vi "Prepare Two Step Build.vi"(8 "error in (no error)":errorcluster, 11 "SDIST in":refnum<class "NI_AB_API_SDIST.lvclass">) -> (0 "error out":errorcluster, 2 "Build Context":refnum<vi>, 3 "SDIST out":refnum<class "NI_AB_API_SDIST.lvclass">)   [LabVIEW 2020, in "NI_AB_API_SDIST.lvclass"]
uses:
  <vilib>/AppBuilder/AB_API/SDIST/NI_AB_API_SDIST.lvclass
  <vilib>/AppBuilder/AB_API/Build/NI_AB_API_Build.lvclass
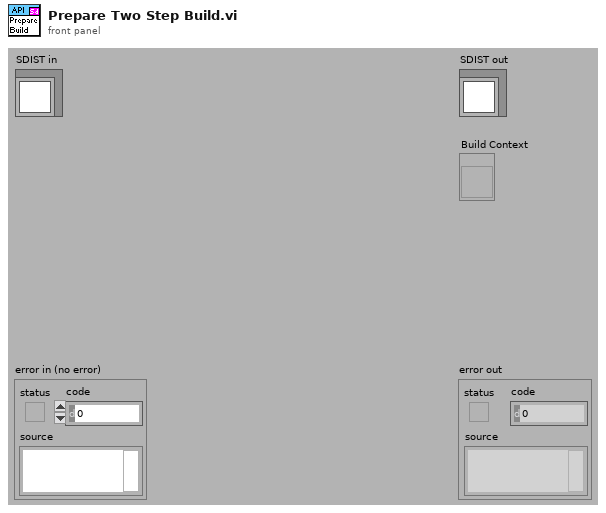
[diagram p1: front panel]
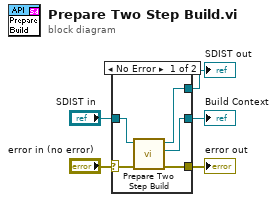
[diagram p0: block diagram]
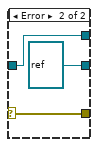
[diagram p2: hidden frame]
diagram:
  n1 = case shown="No Error" "error in (no error)" {
    selector: "error in (no error)" -> [w9 w13]
    tunnel: [w6 w13] -> w4
    tunnel: [w8 w12] -> w2
    tunnel: "SDIST in" -> [w10 w12]
    tunnel: [w7 refnum<vi> refnum ("Build Context")] -> w1
    frame No Error {
      n2 = call-parent "Prepare Two Step Build.vi"("error in (no error)"=w9, "NI_AB_API_Build in"=w10) -> ("error out"=w6:errorcluster, "Build Context"=w7:refnum<vi>, "NI_AB_API_Build out"=w8:refnum<class "NI_AB_API_SDIST.lvclass">)  [unwired: 7 in]
    }
    frame Error {
    }
  }
  "error out" <- w4
  "SDIST out" <- w2
  "Build Context" <- w1
